vi "Read Exception Status.vi"(8 "error in":errorcluster, 11 "device data model in":refnum<class "Device Data Model.lvclass">) -> (0 "error out":errorcluster, 2 "exception status":u8, 3 "device data model out":refnum<class "Device Data Model.lvclass">)   [LabVIEW 2015, in "Modbus Library.lvlib" / "Device Data Model.lvclass"]
doc: "Reads any exception status set in the device model. The exeption status is a single 8-bit integer."
uses:
  Device Data Model.lvclass
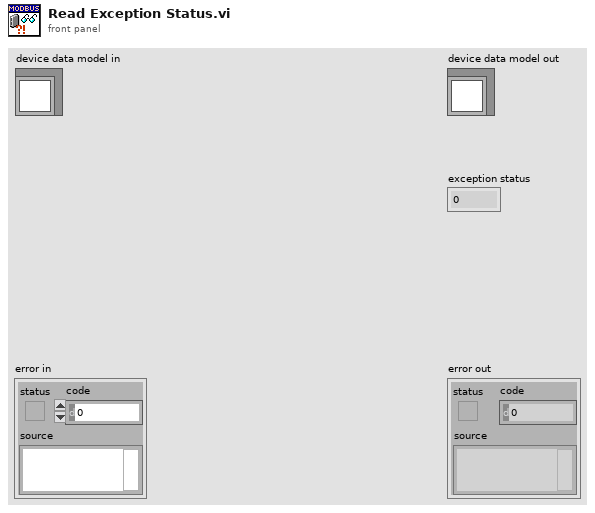
[diagram p1: front panel]
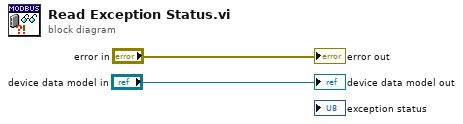
[diagram p0: block diagram]
diagram:
  "error out" <- "error in"
  "device data model out" <- "device data model in"
